vi "Dialog Panel.vi"(8 "error in (no error)":errorcluster, 11 "Dialog":refnum<class "ScriptDialog.lvclass">) -> (0 "error out":errorcluster, 3 "ToolLauncher out":refnum<class "ScriptDialog.lvclass">)   [LabVIEW 2015, in "ScriptDialog.lvclass"]
uses:
  ScriptDialog.lvclass
  _Database/Database.lvclass
  Type Definitiions/Dialog Main ctls and VI ref.ctl
  ScriptDialog.lvclass/ScriptDialog.ctl
  <vilib>/Utility/error.llb/Error Cluster From Error Code.vi
  <vilib>/ErrorRing/Error Ring.xnode
panel:
  in  "Search Contents":string
  in  "Search Results":string
  in  "Tools":cluster{"Configure":bool, "Help":bool}
  in  "Stop":bool
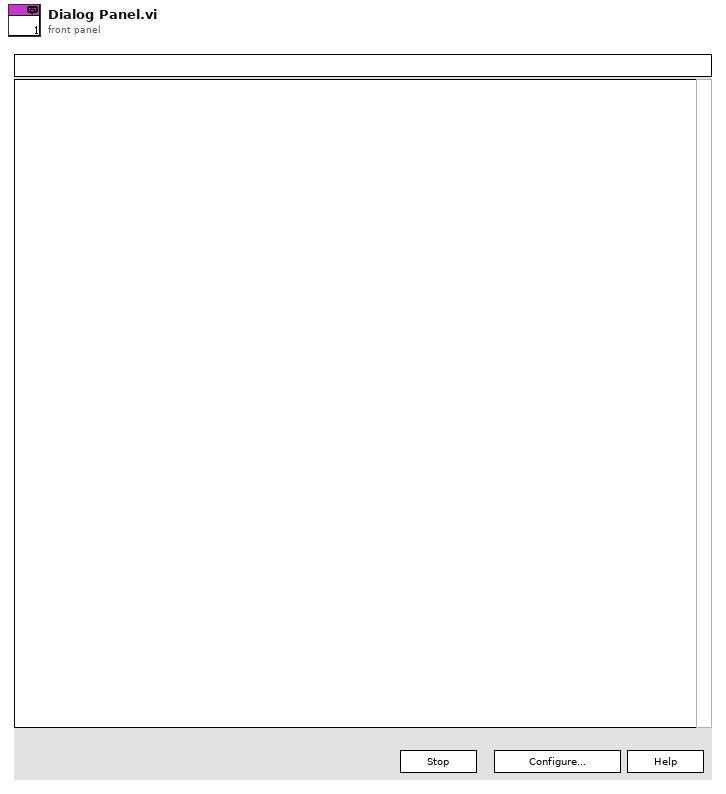
[diagram p1: front panel]
types:
  T1 = typedef "ScriptDialog.lvclass/Dialog Main ctls and VI ref.ctl" = cluster{"Search Results":refnum<vi>, "Search Contents":refnum<vi>, "Stop":refnum<vi>, "Help":refnum<vi>, "Configure":refnum<vi>, "Tools ":refnum<vi>, "Pane 2":refnum<vi>, "Splitter 2":refnum<vi>, "This VI":refnum<vi>}
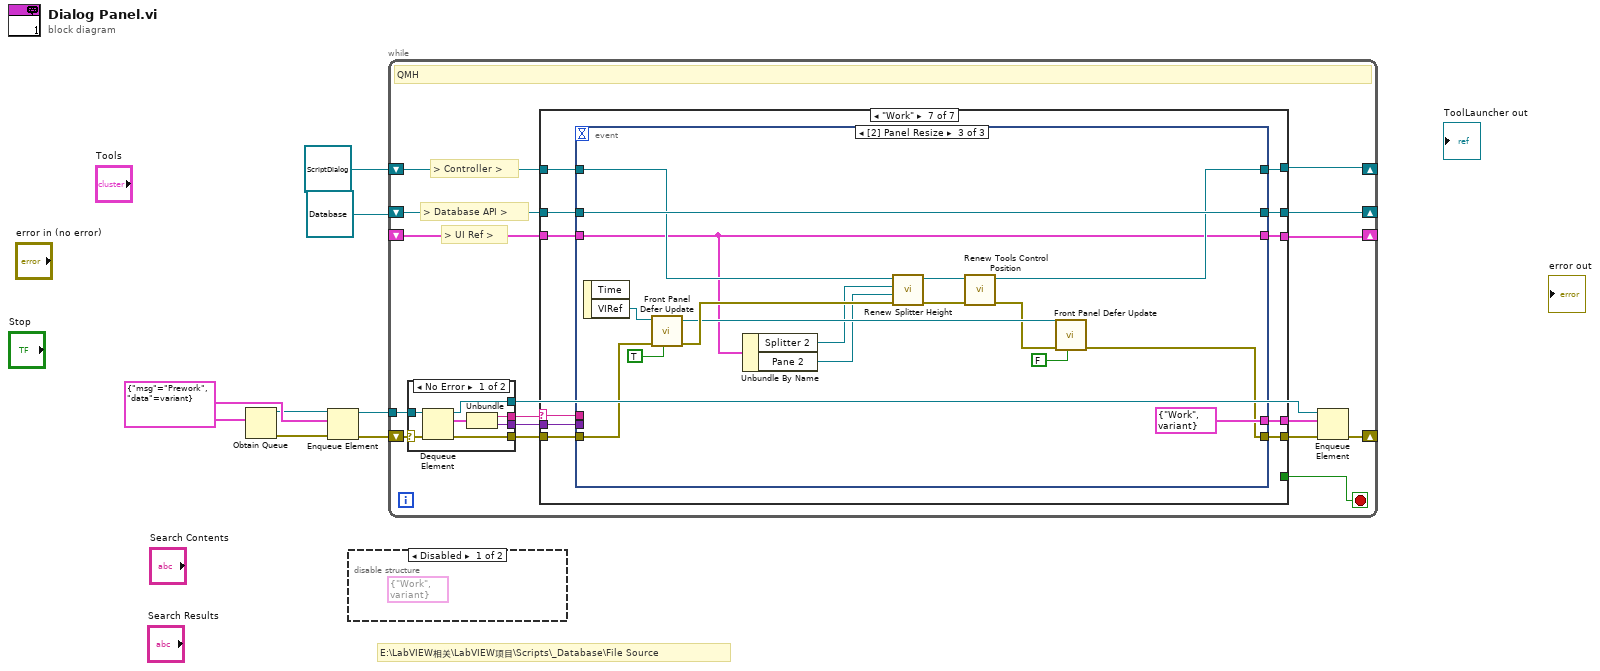
[diagram p0: block diagram]
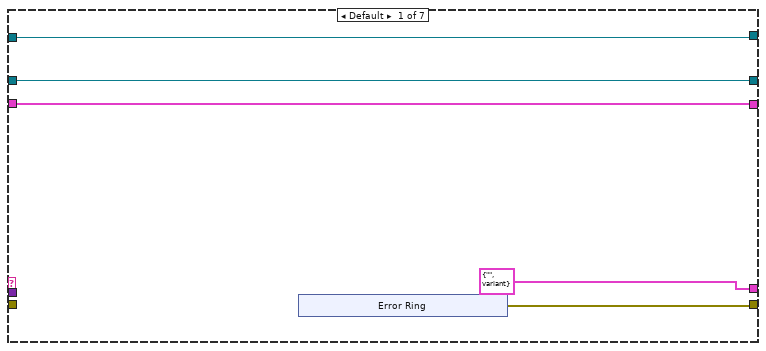
[diagram p3: hidden frame]
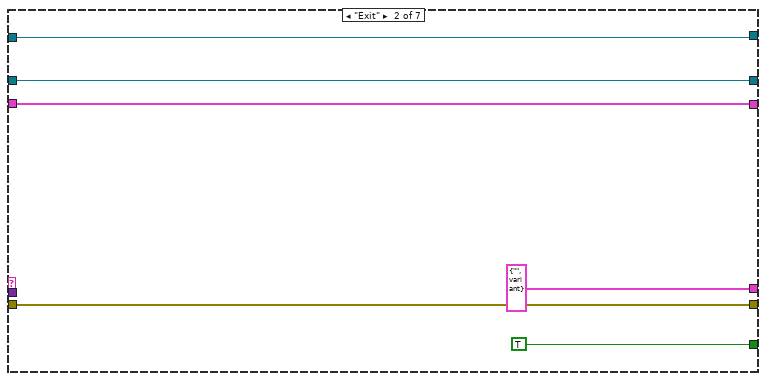
[diagram p4: hidden frame]
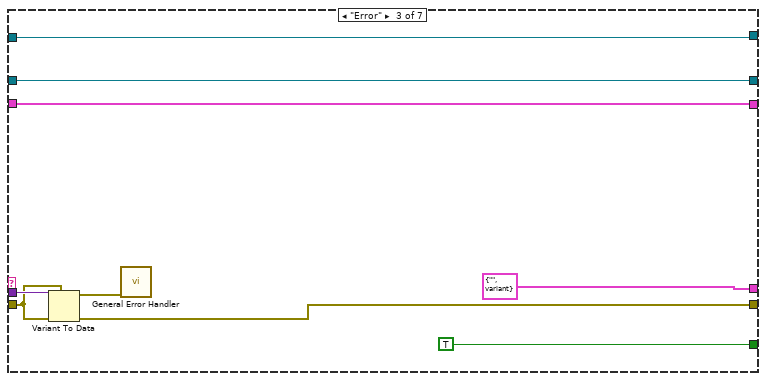
[diagram p5: hidden frame]
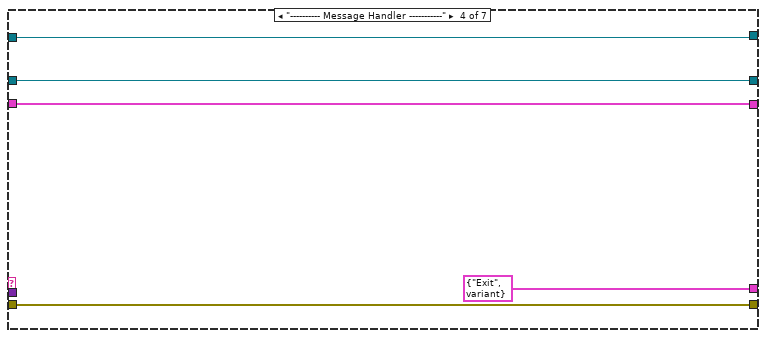
[diagram p6: hidden frame]
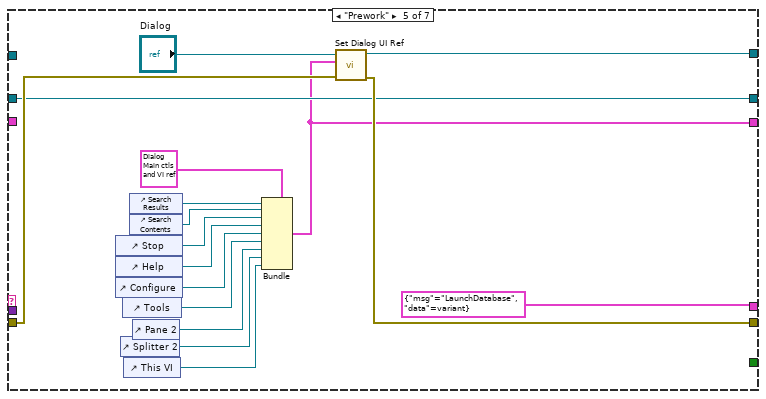
[diagram p7: hidden frame]
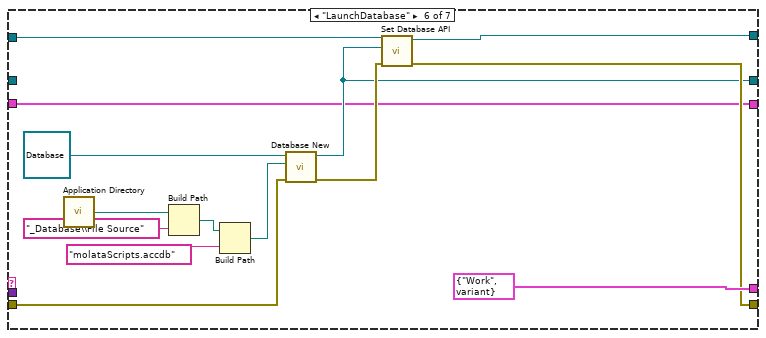
[diagram p8: hidden frame]
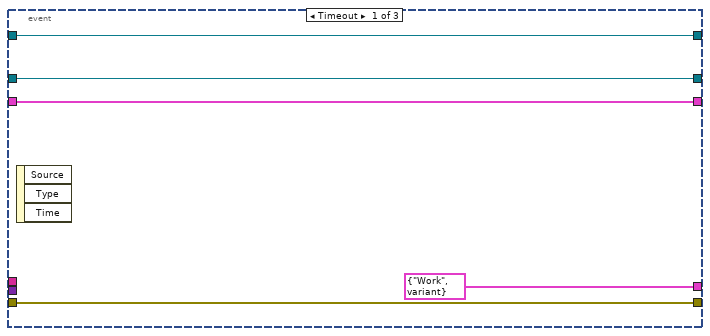
[diagram p9: hidden frame]
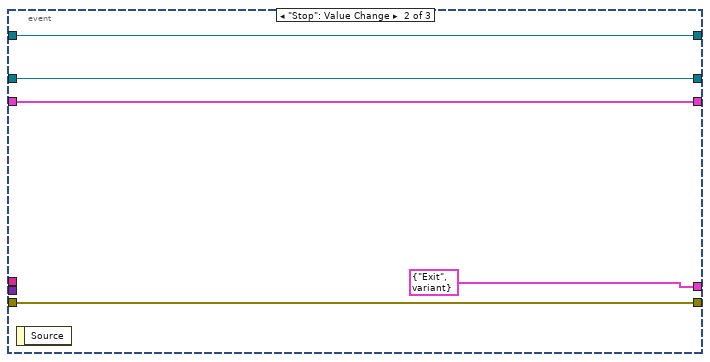
[diagram p10: hidden frame]
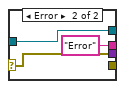
[diagram p11: hidden frame]
diagram:
  w5 = cluster{"msg":string, "data":variant} {"msg"="Prework", "data"=variant}
  # "E:\\LabVIEW相关\\LabVIEW项目\\Scripts\\_Database\\File Source"
  n1 = Obtain Queue(element data type=w5) -> (queue out=w3:refnum<queue>, error out=w4:errorcluster)  [unwired: 4 in, 1 out]
  n2 = Enqueue Element(queue=w3, element=w5, error in (no error)=w4) -> (queue out=w6:refnum<queue>, error out=w7:errorcluster)  [unwired: 1 in, 1 out]
  n3 = disable-structure shown="Disabled" {
    frame Disabled {
      (unwired) cluster{"msg":string, "data":variant} {"msg"="Work", "data"=variant}
    }
    frame Enabled {
    }
  }
  n4 = while {
    tunnel: w6 -> [w22]
    shift-right: [w17] -> _
    shift-left: w7 -> [w23]
    shift-right: [w12] -> _
    shift-left: refnum<class "ScriptDialog.lvclass"> refnum ("ScriptDialog out") -> [w13]
    shift-right: [w11] -> _
    shift-left: refnum<class "Database.lvclass"> refnum ("object out") -> [w10]
    shift-right: [w9] -> _
    shift-left: _ -> [w8]
    stop <- w14 stop-if-true
    # "> UI Ref >"
    # "> Database API >"
    # "> Controller >"
    # "QMH"
    n5 = case shown="No Error" w23 {
      selector: w23 -> [w128 w132]
      tunnel: w22 -> [w129 w130]
      tunnel: [w127 _] -> w21
      tunnel: [w125 "Error" ("msg")] -> w20
      tunnel: [w124 w132] -> w19
      tunnel: [w123 w130] -> w16
      frame No Error {
        n6 = Dequeue Element(queue=w129, error in (no error)=w128) -> (queue out=w123:refnum<queue>, element=w126:cluster{"msg":string, "data":variant}, error out=w127:errorcluster)  [unwired: 1 in, 1 out]
        n7 = Unbundle(w126) -> ("msg"=w125:string, "data"=w124:variant)
      }
      frame Error {
      }
    }
    n8 = case shown="\"Work\"" w20 {
      selector: w20 -> [_ _ _ _ _ _ w93]
      tunnel: w21 -> [_ w39 w47 w53 w63 w78 w95]
      tunnel: w19 -> [_ _ w48 _ _ _ w94]
      tunnel: [w28 w39 w45 w53 w62 w74 w92] -> w18
      tunnel: [cluster{"msg":string, "data":variant} {"msg"="", "data"=variant} cluster{"msg":string, "data":variant} {"msg"="", "data"=variant} cluster{"msg":string, "data":variant} {"msg"="", "data"=variant} cluster{"msg":string, "data":variant} {"msg"="Exit", "data"=variant} cluster{"msg":string, "data":variant} {"msg"="LaunchDatabase", "data"=variant} cluster{"msg":string, "data":variant} {"msg"="Work", "data"=variant} w91] -> w15
      tunnel: [_ TRUE TRUE _ _ _ _] -> w14
      tunnel: w13 -> [w25 w35 w41 w50 _ w76 w90]
      tunnel: [w25 w35 w41 w50 w61 w73 w88] -> w12
      tunnel: [w26 w36 w42 w51 w59 w72 w87] -> w11
      tunnel: w10 -> [w26 w36 w42 w51 w59 _ w89]
      tunnel: [w24 w34 w40 w49 w58 w71 w85] -> w9
      tunnel: w8 -> [w24 w34 w40 w49 _ w71 w86]
      frame Default {
        n9 = xnode "Error Ring"() -> ("error out"=w28:errorcluster)
      }
      frame "Exit" {
      }
      frame "Error" {
        n10 = Variant To Data(error in=w47, type=w47, Variant=w48) -> (data=w46:errorcluster, error out=w45:errorcluster)
        n11 = call <vilib>:"General Error Handler.vi"("error in (no error)"=w46) -> ()  [unwired: 10 in, 5 out]
      }
      frame "---------- Message Handler -----------" {
      }
      frame "Prework" {
        n12 = control-ref of="Stop"() -> (w67:refnum<vi>)
        n13 = control-ref of="Help"() -> (w66:refnum<vi>)
        n14 = control-ref of="Configure"() -> (w65:refnum<vi>)
        n15 = control-ref of="Splitter 2"() -> (w55:refnum<vi>)
        n16 = control-ref of="Tools"() -> (w57:refnum<vi>)
        n17 = control-ref of="This VI"() -> (w54:refnum<vi>)
        n18 = control-ref of="Search Results"() -> (w69:refnum<vi>)
        n19 = control-ref of="Search Contents"() -> (w68:refnum<vi>)
        n20 = control-ref of="Pane 2"() -> (w56:refnum<vi>)
        n21 = Bundle(cluster=T1 {"Search Results"=refnum, "Search Contents"=refnum, "Stop"=refnum, "Help"=refnum, "Configure"=refnum, "Tools "=refnum, "Pane 2"=refnum, "Splitter 2"=refnum, "This VI"=refnum}, "Search Results"=w69, "Search Contents"=w68, "Stop"=w67, "Help"=w66, "Configure"=w65, "Tools"=w57, "Pane 2"=w56, "Splitter 2"=w55, "This VI"=w54) -> (w58:T1)
        n22 = call "Set Dialog UI Ref.vi"("error in (no error)"=w63, "Main ctls and VI ref"=w58, "ScriptDialog in"="Dialog") -> ("error out"=w62:errorcluster, "ScriptDialog out"=w61:refnum<class "ScriptDialog.lvclass">)  [unwired: 7 in]
      }
      frame "LaunchDatabase" {
        n23 = call <vilib>:"Application Directory.vi"() -> ("Application Directory"=w83:path)
        n24 = Build Path(base path=w83, name or relative path="_Database\\File Source") -> (appended path=w81:path)
        n25 = Build Path(base path=w81, name or relative path="molataScripts.accdb") -> (appended path=w79:path)
        n26 = call "Database New.vi"("error in (no error)"=w78, "Database File Path"=w79, "object in"=refnum<class "Database.lvclass"> refnum ("Database")) -> ("error out"=w75:errorcluster, "object out"=w72:refnum<class "Database.lvclass">)  [unwired: 7 in]
        n27 = call "Set Database API.vi"("error in (no error)"=w75, "Database"=w72, "ScriptDialog in"=w76) -> ("error out"=w74:errorcluster, "ScriptDialog out"=w73:refnum<class "ScriptDialog.lvclass">)  [unwired: 7 in]
      }
      frame "Work" {
        n28 = event shown="[2] Panel Resize" {
          selector: _ -> [_ _ _]
          dyn-events: _ -> [_ _ _]
          timeout: _ -> [_ _ _]
          tunnel: w95 -> [w100 w105 w116]
          tunnel: w94 -> [_ _ _]
          tunnel: w93 -> [_ _ _]
          tunnel: [w100 w105 w110] -> w92
          tunnel: [cluster{"msg":string, "data":variant} {"msg"="Work", "data"=variant} cluster{"msg":string, "data":variant} {"msg"="Exit", "data"=variant} cluster{"msg":string, "data":variant} {"msg"="Work", "data"=variant}] -> w91
          tunnel: w90 -> [w98 w103 w118]
          tunnel: w89 -> [w97 w102 w121]
          tunnel: [w98 w103 w114] -> w88
          tunnel: [w97 w102 w121] -> w87
          tunnel: w86 -> [w96 w101 w109]
          tunnel: [w96 w101 w109] -> w85
          event Timeout {
            n29 = event-data() -> ()  [unwired: 1 in, 3 out]
          }
          event "Stop": Value Change {
            n30 = event-data() -> ()  [unwired: 1 in, 1 out]
          }
          event Panel Resize {
            n31 = event-data() -> ("VIRef"=w117:refnum<vi>)  [unwired: 1 in, 1 out]
            n32 = call <userlib>:"Front Panel Defer Update.vi"("Defer Panel Updates(False)"=TRUE, "error in (no error)"=w116, "This VI"=w117) -> ("error out"=w115:errorcluster, "This VI Out"=w112:refnum<vi>)  [unwired: 7 in]
            n33 = Unbundle By Name(w109) -> ("Splitter 2"=w108:refnum<vi>, "Pane 2"=w107:refnum<vi>)
            n34 = call "Renew Splitter Height.vi"("error in (no error)"=w115, "Pane Ref"=w107, "Splitter Ref"=w108, "ScriptDialog.lvclass"=w118) -> ("error out"=w119:errorcluster, "ScriptDialog.lvclass Out"=w120:refnum<class "ScriptDialog.lvclass">)  [unwired: 6 in]
            n35 = call "Renew Tools Control Position.vi"("error in (no error)"=w119, "ScriptDialog"=w120) -> ("error out"=w111:errorcluster, "ScriptDialog  Out"=w114:refnum<class "ScriptDialog.lvclass">)  [unwired: 8 in]
            n36 = call <userlib>:"Front Panel Defer Update.vi"("Defer Panel Updates(False)"=FALSE, "error in (no error)"=w111, "This VI"=w112) -> ("error out"=w110:errorcluster)  [unwired: 7 in, 1 out]
          }
        }
      }
    }
    n37 = Enqueue Element(queue=w16, element=w15, error in (no error)=w18) -> (error out=w17:errorcluster)  [unwired: 1 in, 2 out]
  }
